vi "template action editor UI.vi"(8 "error in (no error)":errorcluster, 10 "user event":refnum<user-event>, 11 "action configuration in":refnum<class "action configuration.lvclass">) -> (0 "error out":errorcluster, 3 "action configuration out":refnum<class "action configuration.lvclass">)   [LabVIEW 2014]
uses:
  <vilib>/NI/TBM Modules/Sequencer/sequencer parent classes/action configuration parent/action configuration.lvclass
  <vilib>/NI/TBM Modules/Sequencer/editor node/user event typedef.ctl
  configuration/configuration data.ctl
  configuration/Template Action Cfg.lvclass
  configuration/Template Action Cfg.lvclass/Template Action Cfg.ctl
  configuration/Write Config. Data.vi
  configuration/Read Config. Data.vi
  <vilib>/NI/TBM Modules/Sequencer/editor node/Simple Sequencer TBM editor node.lvclass
panel:
  in  "Config. Data":T1
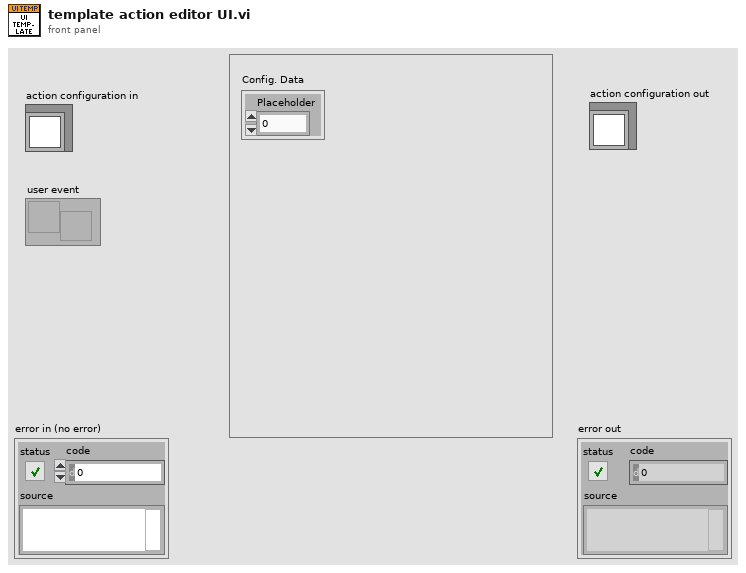
[diagram p1: front panel]
types:
  T1 = typedef "Template Action Cfg.lvclass/configuration data.ctl" = cluster{"Placeholder":dbl}
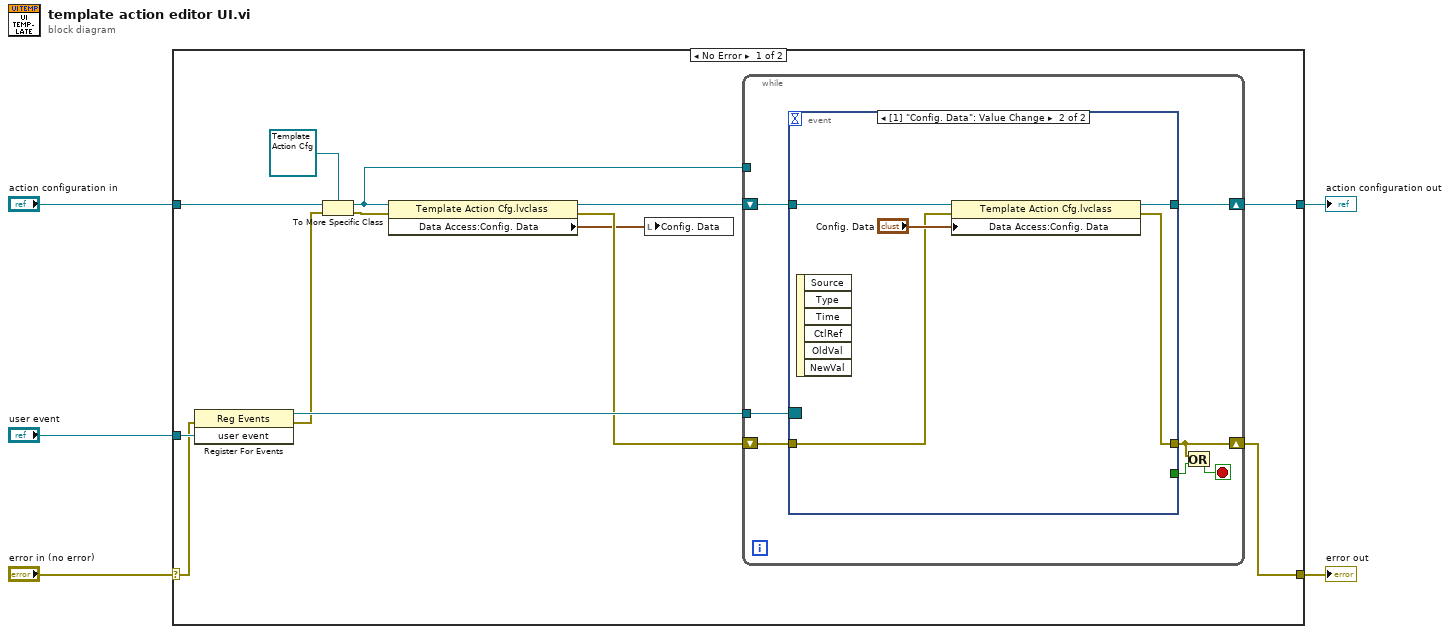
[diagram p0: block diagram]
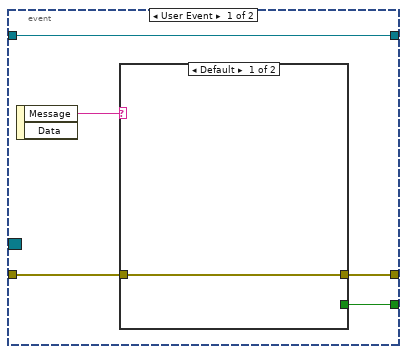
[diagram p2: hidden frame]
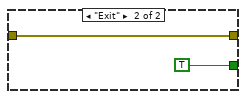
[diagram p3: hidden frame]
diagram:
  n1 = case shown="No Error" "error in (no error)" {
    selector: "error in (no error)" -> [w16 w40]
    tunnel: "user event" -> [w18 _]
    tunnel: "action configuration in" -> [w12 w39]
    tunnel: [w15 w39] -> w2
    tunnel: [w13 w40] -> w1
    frame No Error {
      n2 = register-events(error in=w16, w18) -> (reference out=w17:refnum<event-registration>, error out=w14:errorcluster)  [unwired: 1 in]
      n3 = To More Specific Class(target class=refnum<class "Template Action Cfg.lvclass"> refnum ("Template Action.lvlib:Template Action Config.lvclass"), reference=w12, error in=w14) -> (specific class reference=w11:refnum<class "Template Action Cfg.lvclass">, error out=w9:errorcluster)
      n4 = property class="Template Action Cfg.lvclass"(reference=w11, error in=w9) -> (reference out=w10:refnum<class "Template Action Cfg.lvclass">, error out=w8:errorcluster, "Data Access:Config. Data"=w7:T1)
      n5 = local write "Config. Data"(w7) -> ()
      n6 = while {
        tunnel: w17 -> [w25]
        shift-right: [w23] -> w15
        shift-left: w10 -> [w24]
        tunnel: w11 -> [_]
        shift-right: [w21] -> w13
        shift-left: w8 -> [w22]
        stop <- w19 stop-if-true
        n7 = event shown="[1] \"Config. Data\": Value Change" {
          selector: w25 -> [_ _]
          dyn-events: _ -> [_ _]
          timeout: _ -> [_ _]
          tunnel: [w29 _] -> w20
          tunnel: w24 -> [w28 w38]
          tunnel: [w28 w37] -> w23
          tunnel: w22 -> [w27 w35]
          tunnel: [w26 w34] -> w21
          event User Event {
            n8 = event-data() -> ("Message"=w30:string)  [unwired: 1 in, 1 out]
            n9 = case shown="Default" w30 {
              tunnel: [_ TRUE] -> w29
              tunnel: w27 -> [w31 w32]
              tunnel: [w31 w32] -> w26
              frame Default {
              }
              frame "Exit" {
              }
            }
          }
          event Value Change {
            n10 = event-data() -> ()  [unwired: 1 in, 6 out]
            n11 = property class="Template Action Cfg.lvclass"(reference=w38, error in=w35, "Data Access:Config. Data"="Config. Data") -> (reference out=w37:refnum<class "Template Action Cfg.lvclass">, error out=w34:errorcluster)
          }
        }
        n12 = Or(x=w21, y=w20) -> (x .or. y?=w19:bool)
      }
    }
    frame Error {
    }
  }
  "action configuration out" <- w2
  "error out" <- w1
